vi "GEA2 Script_Determine LED.vi"(0 "LED Data In":string="00 20 08 00 00 00 00 20 40 3D 00 00 00 00", 7 "Match Substring In":string, 11 "Error In":errorcluster) -> (4 "Pass/Fail?":bool, 6 "Report Text":string, 15 "Error Out":errorcluster)   [LabVIEW 2014]
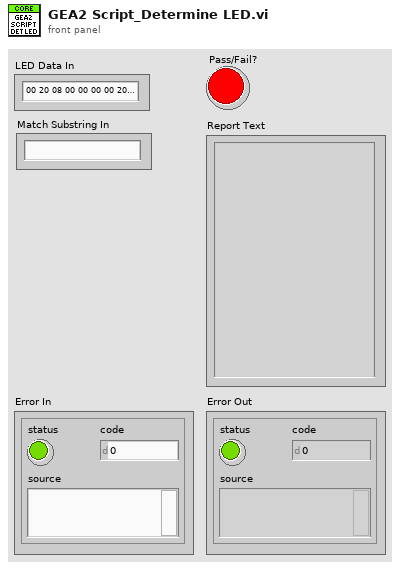
[diagram p1: front panel]
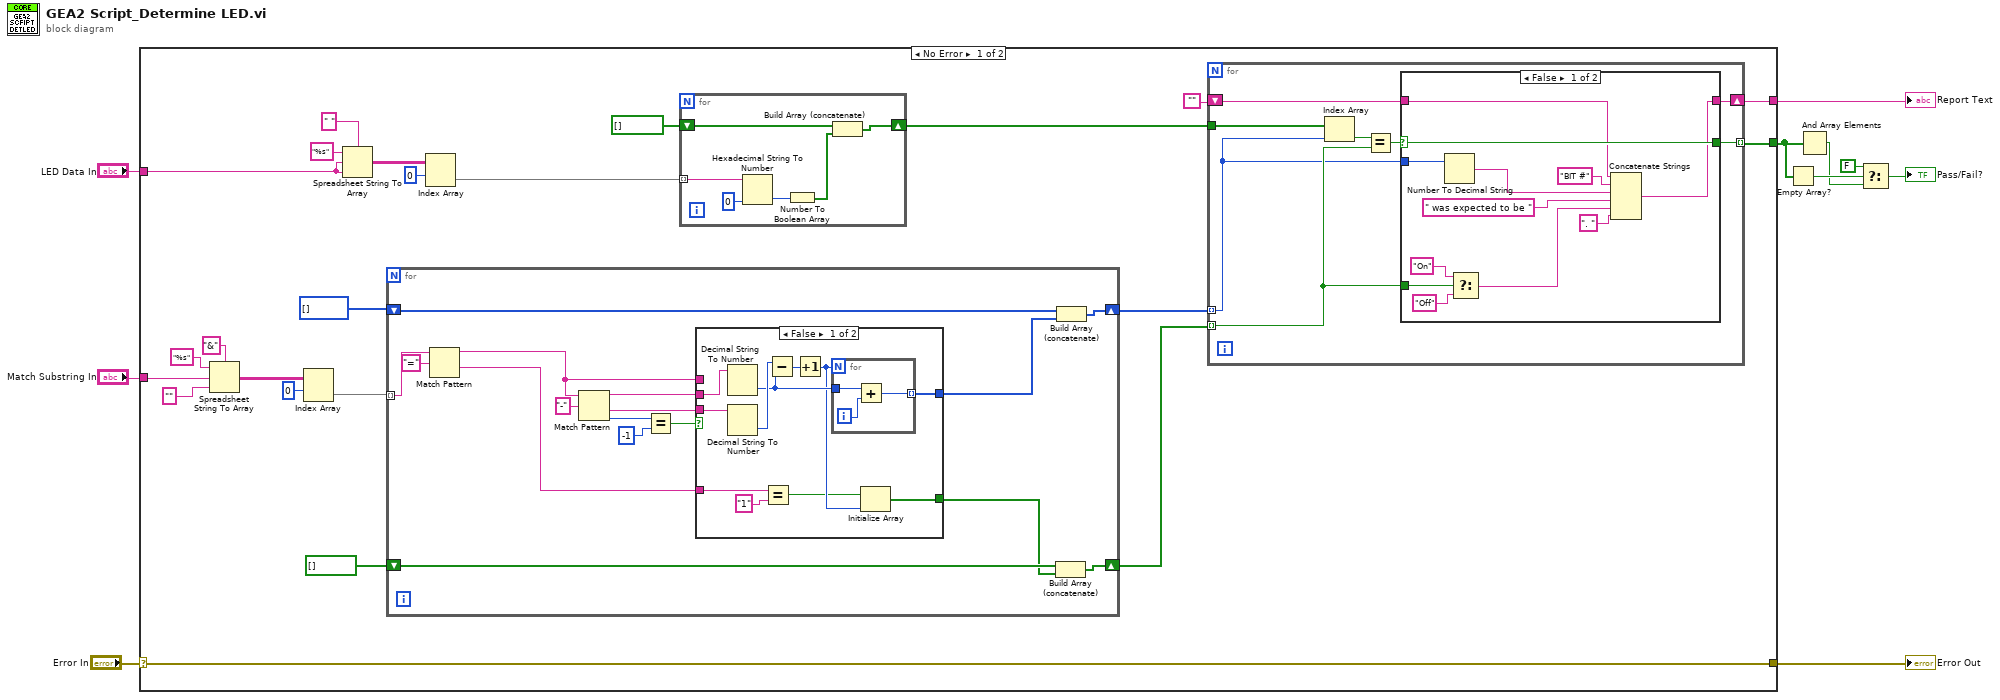
[diagram p0: block diagram]
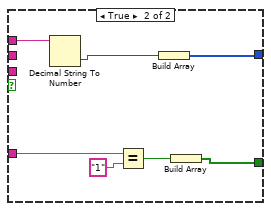
[diagram p3: hidden frame]
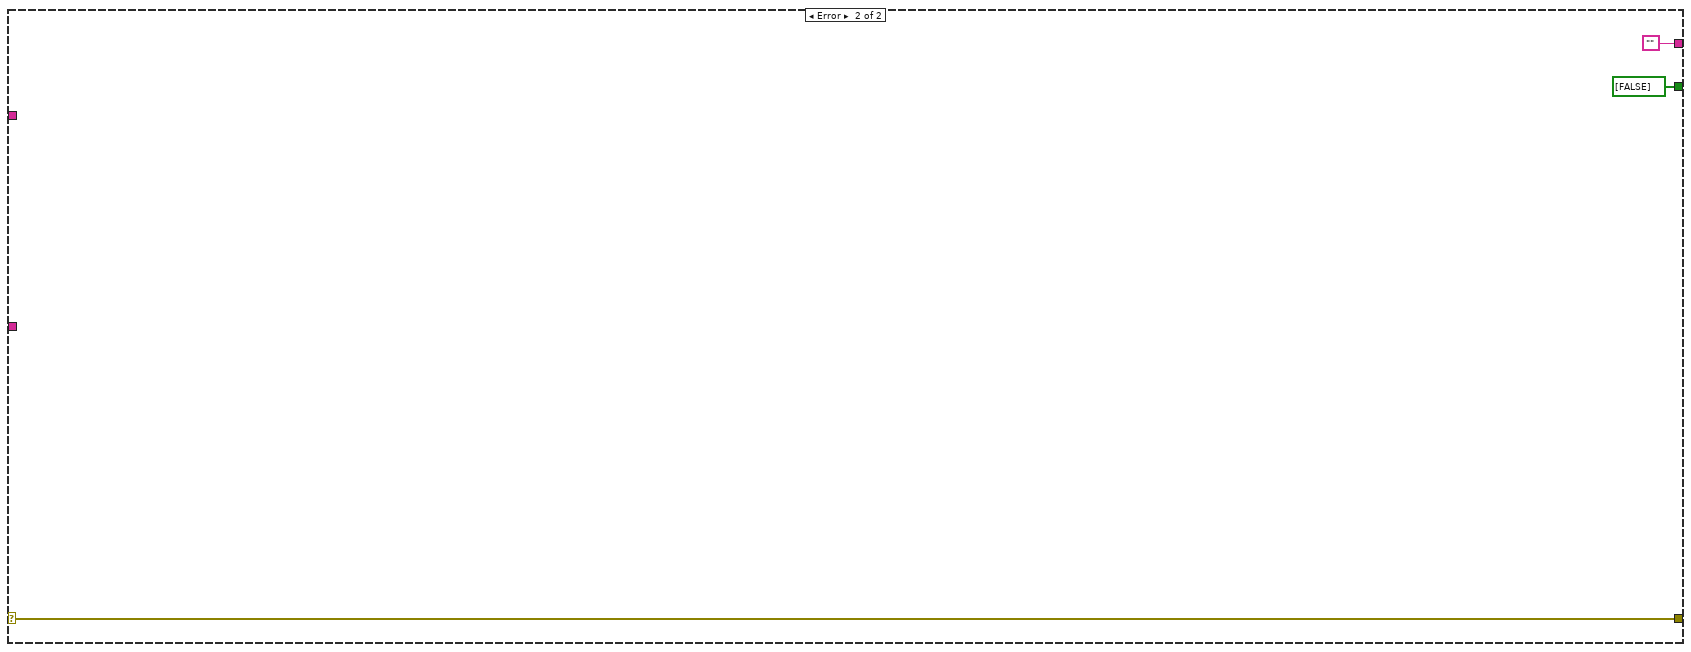
[diagram p4: hidden frame]
diagram:
  n1 = case shown="No Error" "Error In" {
    selector: "Error In" -> [w18 w101]
    tunnel: "LED Data In" -> [w29 _]
    tunnel: "Match Substring In" -> [w19 _]
    tunnel: [w18 w101] -> w7
    tunnel: [w14 ""] -> w6
    tunnel: [w12 bool[] [FALSE]] -> w5
    frame No Error {
      n2 = Spreadsheet String To Array(delimiter (Tab)="&", format string="%s", spreadsheet string=w19, array type (2D Dbl)="") -> (array=w24:string[][])
      n3 = Index Array(array=w24, index (row)=0) -> (element=w22:string[])  [unwired: 1 in]
      n4 = Spreadsheet String To Array(delimiter (Tab)=" ", format string="%s", spreadsheet string=w29, array type (2D Dbl)=w29) -> (array=w31:string[][])
      n5 = for {
        tunnel: w22 -> [w63] mode=indexing
        shift-right: [w65] -> w17
        shift-left: i32[] [] -> [w64]
        shift-right: [w56] -> w16
        shift-left: bool[] [] -> [w58]
        n6 = Match Pattern(string=w63, regular expression="=") -> (before substring=w61:string, after substring=w59:string)  [unwired: 1 in, 2 out]
        n7 = Match Pattern(string=w61, regular expression="-") -> (before substring=w67:string, after substring=w66:string, offset past match=w70:i32)  [unwired: 1 in, 1 out]
        n8 = Equal?(x=w70, y=-1) -> (x = y?=w68:bool)
        n9 = case shown="False" w68 {
          tunnel: w67 -> [w82 _]
          tunnel: w66 -> [w81 _]
          tunnel: w61 -> [_ w92]
          tunnel: [w78 w90] -> w60
          tunnel: w59 -> [w76 w88]
          tunnel: [w73 w86] -> w57
          frame False {
            n10 = Decimal String To Number(string=w82) -> (number=w79:i32)  [unwired: 2 in, 1 out]
            n11 = Decimal String To Number(string=w81) -> (number=w80:i32)  [unwired: 2 in, 1 out]
            n12 = Equal?(x=w76, y="1") -> (x = y?=w74:bool)
            n13 = Subtract(x=w80, y=w79) -> (x-y=w72:i32)
            n14 = Increment(x=w72) -> (x+1=w75:i32)
            n15 = for {
              N: w75 -> [_]
              tunnel: w79 -> [w85]
              tunnel: [w83] -> w78 mode=indexing
              i -> [w84]
              n16 = Add(x=w85, y=w84) -> (x+y=w83:i32)
            }
            n17 = Initialize Array(w74, w75) -> (w73:bool[])
          }
          frame True {
            n18 = Decimal String To Number(string=w92) -> (number=w91:i32)  [unwired: 2 in, 1 out]
            n19 = Equal?(x=w88, y="1") -> (x = y?=w87:bool)
            n20 = Build Array(w91) -> (w90:i32[])
            n21 = Build Array(w87) -> (w86:bool[])
          }
        }
        n22 = Build Array (concatenate)(w58, w57) -> (w56:bool[])
        n23 = Build Array (concatenate)(w64, w60) -> (w65:i32[])
      }
      n24 = Index Array(array=w31, index (row)=0) -> (element=w11:string[])  [unwired: 1 in]
      n25 = for {
        tunnel: w11 -> [w98] mode=indexing
        shift-right: [w94] -> w15
        shift-left: bool[] [] -> [w96]
        n26 = Hexadecimal String To Number(string=w98, default (0uL)=u8 0) -> (number=w97:u8)  [unwired: 1 in, 1 out]
        n27 = Number To Boolean Array(number=w97) -> (Boolean array=w95:bool[])
        n28 = Build Array (concatenate)(w96, w95) -> (w94:bool[])
      }
      n29 = for {
        tunnel: w17 -> [w34] mode=indexing
        tunnel: w16 -> [w35] mode=indexing
        tunnel: w15 -> [w41]
        shift-right: [w38] -> w14
        shift-left: "" -> [w37]
        tunnel: [w36] -> w12 mode=indexing
        n30 = Index Array(array=w41, index=w34) -> (element=w40:bool)
        n31 = Equal?(x=w40, y=w35) -> (x = y?=w39:bool)
        n32 = case shown="False" w39 {
          selector: w39 -> [w53 w54]
          tunnel: [w43 w55] -> w38
          tunnel: w37 -> [w44 w55]
          tunnel: [w53 w54] -> w36
          tunnel: w34 -> [w52 _]
          tunnel: w35 -> [w51 _]
          frame False {
            n33 = Number To Decimal String(number=w52) -> (decimal integer string=w47:string)  [unwired: 1 in]
            n34 = Select(t="On", s=w51, f="Off") -> (s? t:f=w45:string)
            n35 = Concatenate Strings(w44, "BIT #" ("string"), w47, " was expected to be " ("string"), w45, ". " ("string")) -> (w43:string)
          }
          frame True {
          }
        }
      }
    }
    frame Error {
    }
  }
  "Error Out" <- w7
  "Report Text" <- w6
  n36 = Empty Array?(array=w5) -> (empty?=w4:bool)
  n37 = And Array Elements(Boolean array=w5) -> (logical AND=w3:bool)
  n38 = Select(t=FALSE, s=w4, f=w3) -> (s? t:f=→"Pass/Fail?":bool)
